vi "Delete Channel Name and Error Controls.vi"(0 "vi in":refnum<vi>, 11 "error in":errorcluster) -> (4 "vi out":refnum<vi>, 15 "error out":errorcluster)   [LabVIEW 2021, in "Converter.lvlib"]
uses:
  Converter.lvlib
  <vilib>/Utility/traverseref.llb/TRef TravTarget.ctl
  <vilib>/Utility/traverseref.llb/VI Scripting - Traverse.lvlib
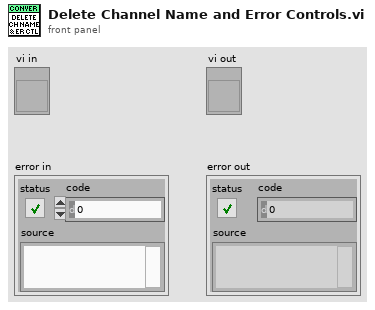
[diagram p1: front panel]
types:
  T1 = typedef "TRef TravTarget.ctl" = enum16{"FP", "BD", "Other"}
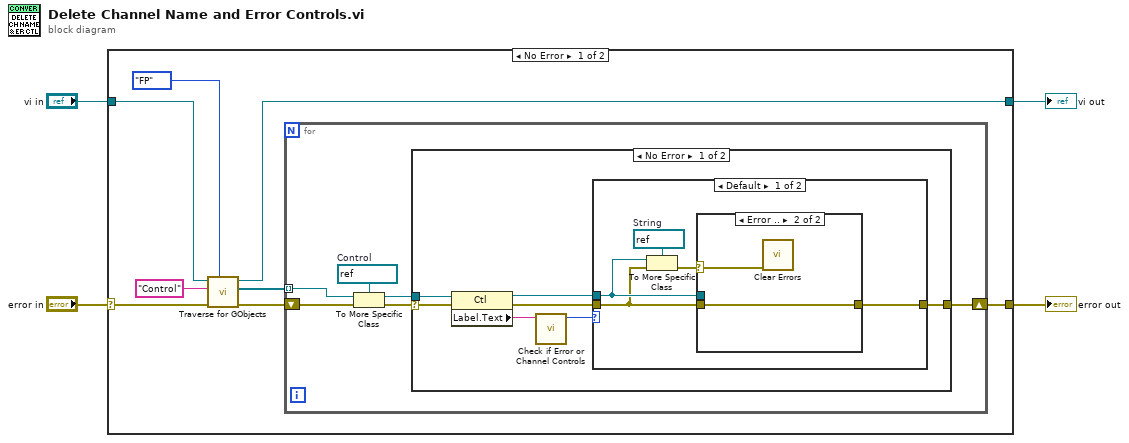
[diagram p0: block diagram]
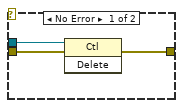
[diagram p2: hidden frame]
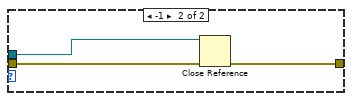
[diagram p3: hidden frame]
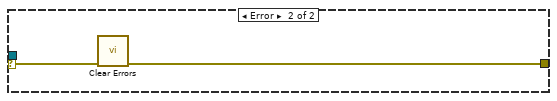
[diagram p4: hidden frame]
diagram:
  n1 = case shown="No Error" "error in" {
    selector: "error in" -> [w7 w41]
    tunnel: [w11 w41] -> w4
    tunnel: [w10 w42] -> w3
    tunnel: "vi in" -> [w6 w42]
    frame No Error {
      n2 = call <vilib>:"Traverse for GObjects.vi"("Traverse Target"=TRef_TravTarget."FP", "error in (no error)"=w7, "Class Name"="Control", "VI Refnum"=w6) -> ("error out"=w8:errorcluster, "References"=w9:refnum<vi>[], "dup VI Refnum"=w10:refnum<vi>)  [unwired: 4 in, 1 out]
      n3 = for {
        tunnel: w9 -> [w18] mode=indexing
        shift-right: [w13] -> w11
        shift-left: w8 -> [w17]
        w16 = refnum<vi> refnum  # Control
        n4 = To More Specific Class(target class=w16, reference=w18, error in=w17) -> (specific class reference=w15:refnum<vi>, error out=w14:errorcluster)
        n5 = case shown="No Error" w14 {
          selector: w14 -> [w24 w40]
          tunnel: w15 -> [w25 _]
          tunnel: [w19 w39] -> w13
          frame No Error {
            n6 = property class="Ctl"(reference=w25, error in=w24) -> (reference out=w20:refnum<vi>, error out=w21:errorcluster, "Label.Text"=w23:string)
            n7 = call "Check if Error or Channel Controls.vi"("label.text"=w23) -> ("offset past match"=w22:i32)  [unwired: 9 in, 1 out]
            n8 = case shown="Default" w22 {
              tunnel: w21 -> [w26 w37]
              tunnel: w20 -> [w28 w36]
              tunnel: [w30 w38] -> w19
              frame Default {
                w29 = refnum<vi> refnum  # String
                n9 = To More Specific Class(target class=w29, reference=w28, error in=w26) -> (error out=w27:errorcluster)  [unwired: 1 out]
                n10 = case shown="Error .." w27 {
                  selector: w27 -> [_ w34]
                  tunnel: w26 -> [w33 w35]
                  tunnel: [w32 w35] -> w30
                  tunnel: w28 -> [w31 _]
                  frame No Error {
                    n11 = invoke class="Ctl" method="Delete"(reference=w31, error in=w33) -> (error out=w32:errorcluster)  [unwired: 1 in, 2 out]
                  }
                  frame Error {
                    n12 = call <vilib>:"Clear Errors.vi"("error in (no error)"=w34) -> ()  [unwired: 5 in, 2 out]
                  }
                }
              }
              frame -1 {
                n13 = Close Reference(reference=w36, error in (no error)=w37) -> (error out=w38:errorcluster)
              }
            }
          }
          frame Error {
            n14 = call <vilib>:"Clear Errors.vi"("error in (no error)"=w40) -> ("error out"=w39:errorcluster)  [unwired: 5 in, 1 out]
          }
        }
      }
    }
    frame Error {
    }
  }
  "error out" <- w4
  "vi out" <- w3
